vi "Wait for Operation Complete.vi"(8 "error in (no error)":errorcluster, 10 "Maximum Time (10000 ms)":u32=10000, 11 "VISA resource name":refnum<visa-resource-name>) -> (0 "error out":errorcluster, 3 "VISA resource name out":refnum<visa-resource-name>)   [LabVIEW 2012, in "Fluke 5080.lvlib"]
doc: "Waits for the current operation to finish. This VI can be used after any operation VIs which could be potentially overlaped."
uses:
  <instrlib>/Fluke 5080/Fluke 5080.lvlib
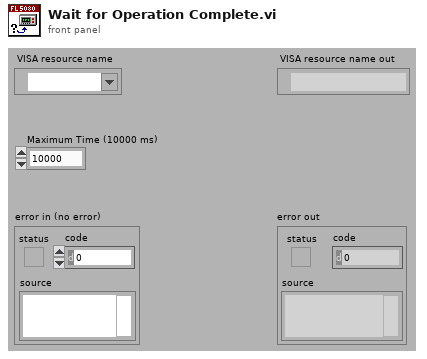
[diagram p1: front panel]
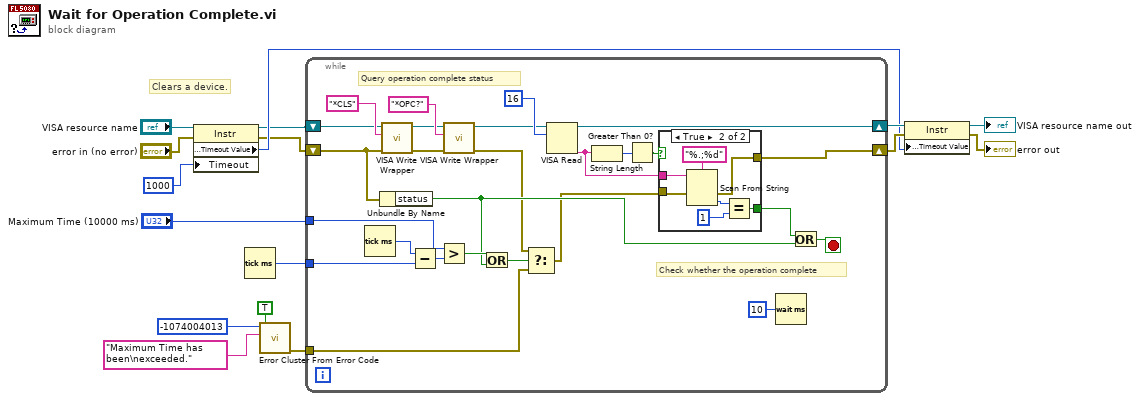
[diagram p0: block diagram]
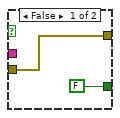
[diagram p2: hidden frame]
diagram:
  # "Clears a device."
  n1 = property class="Instr"(reference="VISA resource name", error in="error in (no error)", "Timeout"=u32 1000 ("General Settings:Timeout Value")) -> (reference out=w2:refnum<visa-resource-name>, error out=w1:errorcluster, "General Settings:Timeout Value"=w4:u32)
  n2 = Tick Count (ms)() -> (millisecond timer value=w16:u32)
  n3 = call <vilib>:"Error Cluster From Error Code.vi"("show call chain? (False)"=TRUE, "error message (\"\")"="Maximum Time has been\nexceeded." ("error message (\"\")"), "error code (0)"=-1074004013) -> ("error out"=w12:errorcluster)  [unwired: 1 in, 5 out]
  n4 = while {
    tunnel: "Maximum Time (10000 ms)" -> [w36]
    tunnel: w16 -> [w39]
    tunnel: w12 -> [w31]
    shift-right: [w38] -> w6
    shift-left: w1 -> [w18]
    shift-right: [w42] -> w8
    shift-left: w2 -> [w20]
    stop <- w37 stop-if-true
    # "Query operation complete status"
    # "Check whether the operation complete"
    n5 = Tick Count (ms)() -> (millisecond timer value=w40:u32)
    n6 = Unbundle By Name(w18) -> ("status"=w32:bool)
    n7 = call <instrlib>:"VISA Write Wrapper.vi"("error in (no error)"=w18, "Write Buffer"="*CLS" ("write buffer"), "VISA resource name"=w20) -> ("error out"=w17:errorcluster, "VISA resource name out"=w19:refnum<visa-resource-name>)  [unwired: 6 in, 1 out]
    n8 = Subtract(x=w40, y=w39) -> (x-y=w35:u32)
    n9 = Greater?(x=w36, y=w35) -> (0:w34:bool)
    n10 = call <instrlib>:"VISA Write Wrapper.vi"("error in (no error)"=w17, "Write Buffer"="*OPC?" ("write buffer"), "VISA resource name"=w19) -> ("error out"=w24:errorcluster, "VISA resource name out"=w23:refnum<visa-resource-name>)  [unwired: 6 in, 1 out]
    n11 = Or(x=w34, y=w32) -> (x .or. y?=w33:bool)
    n12 = Select(t=w24, s=w33, f=w31) -> (s? t:f=w28:errorcluster)
    n13 = VISA Read(VISA resource name=w23, byte count=u32 16) -> (VISA resource name out=w42:refnum<visa-resource-name>, read buffer=w25:string)  [unwired: 1 in, 2 out]
    n14 = String Length(string=w25) -> (length=w27:i32)
    n15 = Greater Than 0?(x=w27) -> (x > 0?=w26:bool)
    n16 = case shown="True" w26 {
      tunnel: [w44 w50] -> w38
      tunnel: [FALSE w47] -> w29
      tunnel: w28 -> [w44 w46]
      tunnel: w25 -> [_ w45]
      frame False {
      }
      frame True {
        n17 = Scan From String(format string="%.;%d", input string=w45, error in=w46) -> (error out=w50:errorcluster, output 1=w49:i32)  [unwired: 1 in, 3 out]
        n18 = Equal?(x=w49, y=1 ("index")) -> (x = y?=w47:bool)
      }
    }
    n19 = Wait (ms)(milliseconds to wait=u32 10) -> ()  [unwired: 1 out]
    n20 = Or(x=w29, y=w32) -> (x .or. y?=w37:bool)
  }
  n21 = property class="Instr"(reference=w8, error in=w6, "General Settings:Timeout Value"=w4) -> (reference out=→"VISA resource name out":refnum<visa-resource-name>, error out=→"error out":errorcluster)
